vi "svx_SC Line Arrow.vi"(4 "shaft rotating direction":u16(ring) items=["CCW", "CW"], 6 "color":u32(colorbox)=10184, 10 "Plot Area:Size":T1, 11 "Picture in":picture) -> (2 "Plot Area:Size out":T1, 3 "new picture":picture)   [LabVIEW 2017, in "SVX SC Line.xctl"]
uses:
  <vilib>/addons/_XControls/Shaft Centerline/SVX SC Line.xctl
  <vilib>/Utility/miscctls.llb/LVBoundsTypeDef.ctl
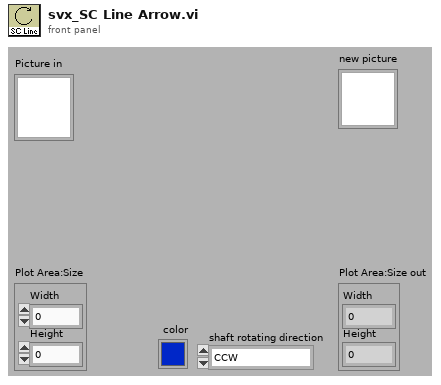
[diagram p1: front panel]
types:
  T1 = typedef "LVBoundsTypeDef.ctl" = cluster{"Width":u32, "Height":u32}
  T2 = cluster{"Width":u16, "Style":enum32{"Solid", "Dash", "Dot", "DashDot", "DashDotDot"}}
  T3 = cluster{"left":i16, "top":i16, "right":i16, "bottom":i16}
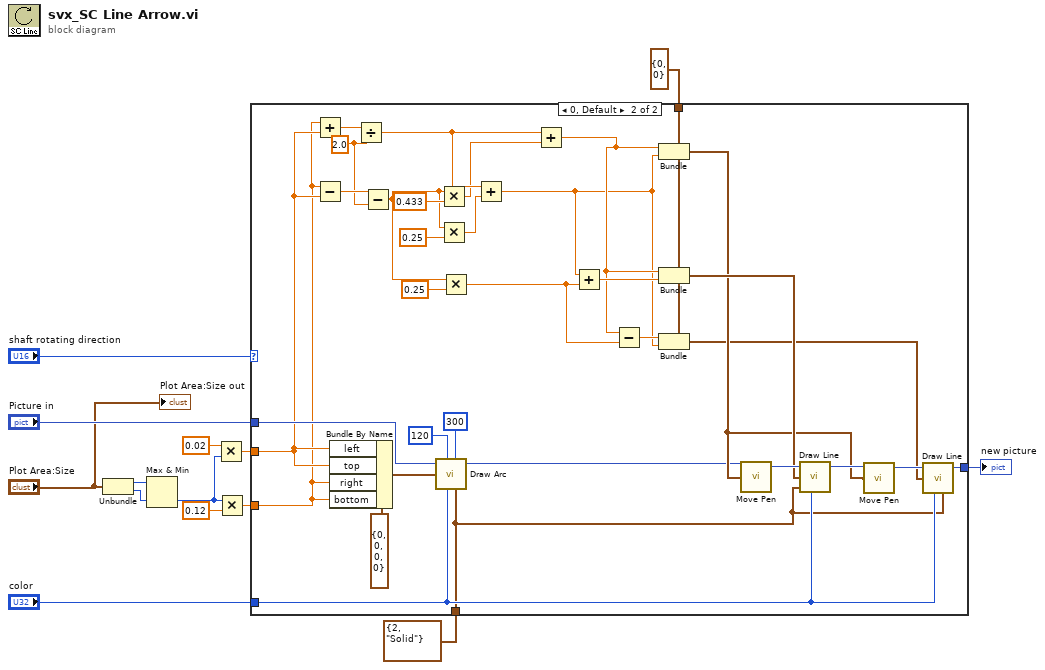
[diagram p0: block diagram]
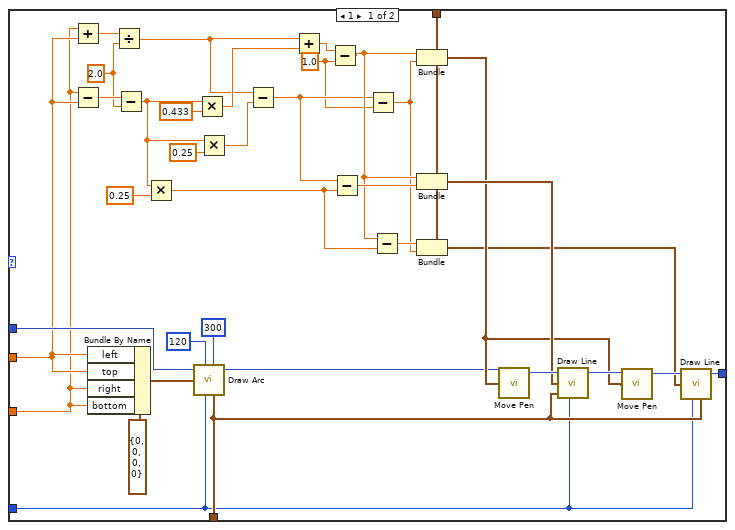
[diagram p2: hidden frame]
diagram:
  n1 = Unbundle("Plot Area:Size") -> ("Width"=w13:u32, "Height"=w12:u32)
  n2 = Max & Min(x=w13, y=w12) -> (min(x,y)=w6:u32)  [unwired: 1 out]
  n3 = Multiply(x=0.02, y=w6) -> (x*y=w8:dbl)
  n4 = Multiply(x=w6, y=0.12) -> (x*y=w9:dbl)
  n5 = case shown="0, Default" "shaft rotating direction" {
    tunnel: "Picture in" -> [w50 w83]
    tunnel: w9 -> [w32 w66]
    tunnel: w8 -> [w45 w78]
    tunnel: [w38 w71] -> w7
    tunnel: T2 {"Width"=2, "Style"=enum."Solid"} ("pen") -> [w36 w57]
    tunnel: "color" -> [w35 w69]
    tunnel: cluster{"x":i16, "y":i16} {"x"=0, "y"=0} ("cluster") -> [w15 w51]
    frame 1 {
      w19 = 1.0 ("y")
      w25 = 2.0 ("y")
      n6 = Add(x=w32, y=w45) -> (x+y=w34:dbl)
      n7 = Subtract(x=w32, y=w45) -> (x-y=w26:dbl)
      n8 = Bundle By Name(cluster=T3 {"left"=0, "top"=0, "right"=0, "bottom"=0} ("rect"), "left"=w45, "top"=w45, "right"=w32, "bottom"=w32) -> (w47:T3)
      n9 = Divide(x=w34, y=w25) -> (x/y=w24:dbl)
      n10 = Subtract(x=w26, y=w25) -> (x-y=w17:dbl)
      n11 = Multiply(x=w17, y=0.25) -> (x*y=w28:dbl)
      n12 = call <vilib>:"Draw Arc.vi"("picture"=w50, "start angle[degrees]"=i16 120, "rect"=w47, "color(black)"=w35, "arc size[degrees]"=i16 300, "pen"=w36) -> ("new picture"=w37:picture)  [unwired: 3 in]
      n13 = Multiply(x=w17, y=0.433) -> (x*y=w30:dbl)
      n14 = Multiply(x=w17, y=0.25) -> (x*y=w16:dbl)
      n15 = Subtract(x=w24, y=w16) -> (x-y=w21:dbl)
      n16 = Add(x=w24, y=w30) -> (x+y=w23:dbl)
      n17 = Subtract(x=w23, y=w19) -> (x-y=w22:dbl)
      n18 = Subtract(x=w21, y=w28) -> (x-y=w29:dbl)
      n19 = Subtract(x=w21, y=w19) -> (x-y=w20:dbl)
      n20 = Subtract(x=w22, y=w28) -> (x-y=w27:dbl)
      n21 = Bundle(cluster=w15, "x"=w22, "y"=w20) -> (w40:cluster{"x":i16, "y":i16})
      n22 = Bundle(cluster=w15, "x"=w22, "y"=w29) -> (w43:cluster{"x":i16, "y":i16})
      n23 = Bundle(cluster=w15, "x"=w27, "y"=w20) -> (w39:cluster{"x":i16, "y":i16})
      n24 = call <vilib>:"Move Pen.vi"("new position"=w40, "picture"=w37) -> ("new picture"=w44:picture)  [unwired: 3 in]
      n25 = call <vilib>:"Draw Line.vi"("picture"=w44, "end point"=w43, "color(black)"=w35, "pen"=w36) -> ("new picture"=w41:picture)  [unwired: 5 in]
      n26 = call <vilib>:"Move Pen.vi"("new position"=w40, "picture"=w41) -> ("new picture"=w42:picture)  [unwired: 3 in]
      n27 = call <vilib>:"Draw Line.vi"("picture"=w42, "end point"=w39, "color(black)"=w35, "pen"=w36) -> ("new picture"=w38:picture)  [unwired: 5 in]
    }
    frame 0, Default {
      w59 = 2.0 ("y")
      n28 = Add(x=w66, y=w78) -> (x+y=w68:dbl)
      n29 = Subtract(x=w66, y=w78) -> (x-y=w60:dbl)
      n30 = Bundle By Name(cluster=T3 {"left"=0, "top"=0, "right"=0, "bottom"=0} ("rect"), "left"=w78, "top"=w78, "right"=w66, "bottom"=w66) -> (w80:T3)
      n31 = Divide(x=w68, y=w59) -> (x/y=w65:dbl)
      n32 = Subtract(x=w60, y=w59) -> (x-y=w54:dbl)
      n33 = call <vilib>:"Draw Arc.vi"("picture"=w83, "start angle[degrees]"=i16 120, "rect"=w80, "color(black)"=w69, "arc size[degrees]"=i16 300, "pen"=w57) -> ("new picture"=w70:picture)  [unwired: 3 in]
      n34 = Multiply(x=w54, y=0.433) -> (x*y=w58:dbl)
      n35 = Multiply(x=w54, y=0.25) -> (x*y=w52:dbl)
      n36 = Multiply(x=w54, y=0.25) -> (x*y=w63:dbl)
      n37 = Add(x=w65, y=w52) -> (x+y=w55:dbl)
      n38 = Add(x=w65, y=w58) -> (x+y=w56:dbl)
      n39 = Add(x=w55, y=w63) -> (x+y=w64:dbl)
      n40 = Subtract(x=w56, y=w63) -> (x-y=w62:dbl)
      n41 = Bundle(cluster=w51, "x"=w56, "y"=w55) -> (w73:cluster{"x":i16, "y":i16})
      n42 = Bundle(cluster=w51, "x"=w56, "y"=w64) -> (w76:cluster{"x":i16, "y":i16})
      n43 = Bundle(cluster=w51, "x"=w62, "y"=w55) -> (w72:cluster{"x":i16, "y":i16})
      n44 = call <vilib>:"Move Pen.vi"("new position"=w73, "picture"=w70) -> ("new picture"=w77:picture)  [unwired: 3 in]
      n45 = call <vilib>:"Draw Line.vi"("picture"=w77, "end point"=w76, "color(black)"=w69, "pen"=w57) -> ("new picture"=w74:picture)  [unwired: 5 in]
      n46 = call <vilib>:"Move Pen.vi"("new position"=w73, "picture"=w74) -> ("new picture"=w75:picture)  [unwired: 3 in]
      n47 = call <vilib>:"Draw Line.vi"("picture"=w75, "end point"=w72, "color(black)"=w69, "pen"=w57) -> ("new picture"=w71:picture)  [unwired: 5 in]
    }
  }
  "new picture" <- w7
  "Plot Area:Size out" <- "Plot Area:Size"
